vi "Event Camera.vi"() -> ()   [LabVIEW 2025]
panel:
  in  "Stop Preview":bool
  out "Image":T1(plugin-control)
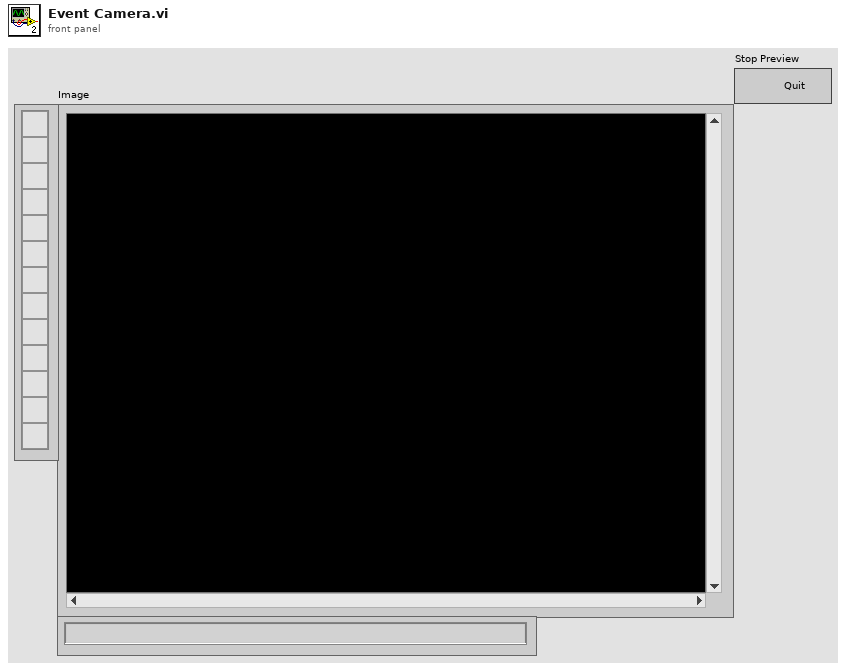
[diagram p1: front panel]
types:
  T1 = typedef "IMAQ Image.ctl" = refnum<image>
  T2 = typedef "Image Type" = u32
  T3 = enum16{"open", "replace", "create", "open or create", "replace or create", "replace or create with confirmation"}
  T4 = enum16{"big-endian, network order", "native, host order", "little-endian"}
  T5 = enum16{"Standard", "Buffered", "CRLF", "Immediate"}
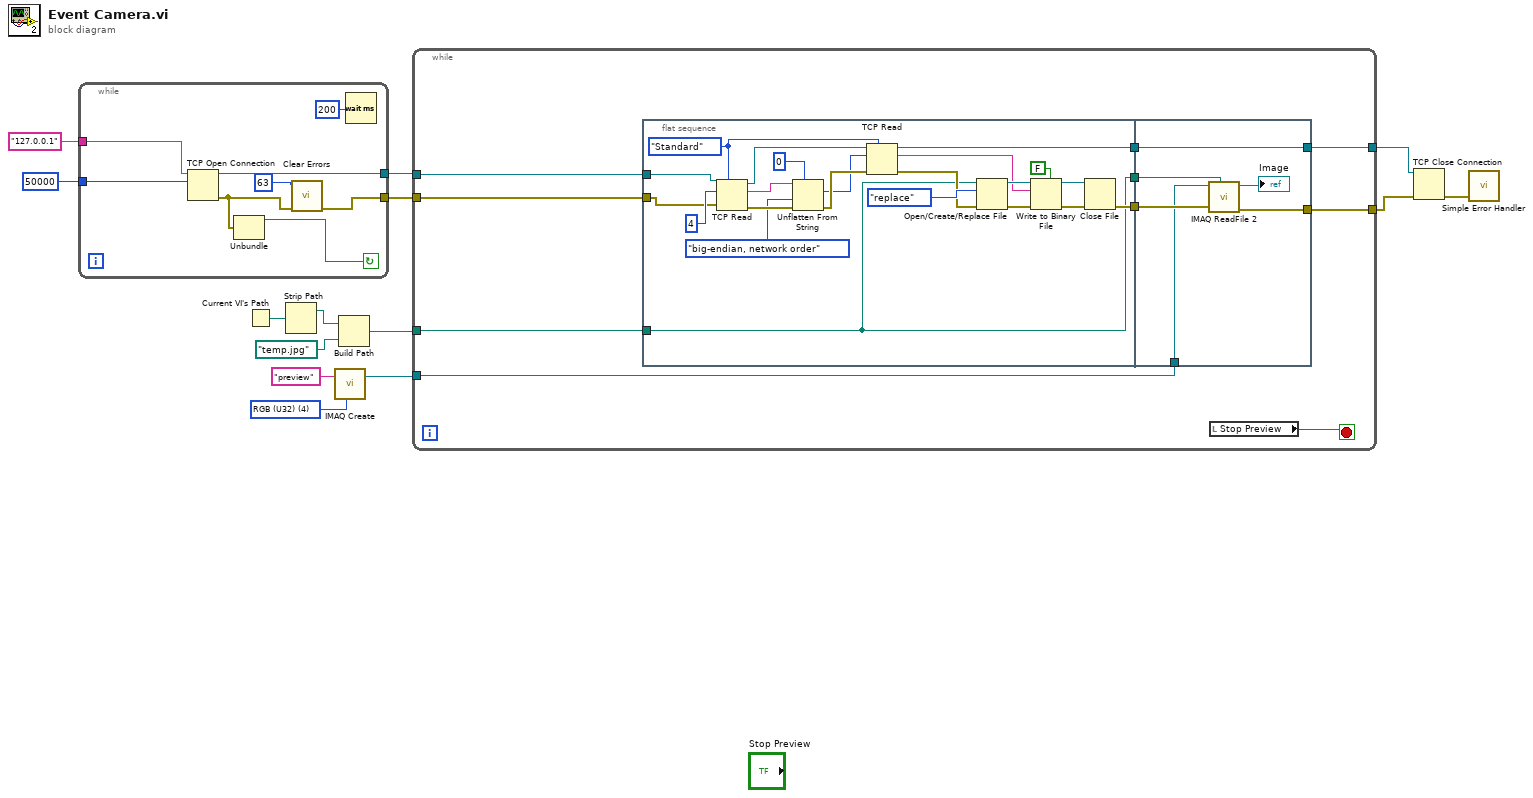
[diagram p0: block diagram]
diagram:
  w10 = T2 4 items=["Grayscale (U8)", "Grayscale (I16)", "Grayscale (SGL)", "Complex (CSG)", "RGB (U32)", "HSL (U32)", "RGB (U64)", "Grayscale (U16)"] ("Image Type")
  n1 = while {
    tunnel: [w19] -> w11
    tunnel: [w22] -> w12
    tunnel: u16 50000 ("remote port or service name") -> [w21]
    tunnel: "127.0.0.1" ("address") -> [w15]
    stop <- w16 continue-if-true
    n2 = TCP Open Connection(address=w15, remote port or service name=w21) -> (connection ID=w22:refnum<k5>, error out=w20:errorcluster)  [unwired: 3 in]
    n3 = Unbundle(w20) -> ("status"=w16:bool)  [unwired: 2 out]
    n4 = call <vilib>:"Clear Errors.vi"("error in (no error)"=w20, "specific error code to clear (0: all)"=63) -> ("error out"=w19:errorcluster)  [unwired: 4 in, 1 out]
    n5 = Wait (ms)(milliseconds to wait=u32 200) -> ()  [unwired: 1 out]
  }
  n6 = Current VI's Path() -> (path=w2:path)
  n7 = Strip Path(path=w2) -> (stripped path=w1:path)  [unwired: 1 out]
  n8 = call "IMAQ Create"("Image Name"="preview", "Image Type"=w10) -> ("New Image"=w6:T1)  [unwired: 3 in, 1 out]
  n9 = Build Path(base path=w1, name or relative path=path "temp.jpg") -> (appended path=w3:path)
  n10 = while {
    tunnel: w6 -> [w27]
    tunnel: [w28] -> w5
    tunnel: [w32] -> w4
    tunnel: w3 -> [w30]
    tunnel: w11 -> [w25]
    tunnel: w12 -> [w24]
    stop <- w23 stop-if-true
    n11 = flat-sequence {
      tunnel: w30 -> [w36]
      tunnel: [w38] -> w31
      tunnel: [w37] -> w29
      tunnel: [w36] -> w26
      tunnel: w25 -> [w34]
      tunnel: w24 -> [w33]
      tunnel: [w60] -> w32
      tunnel: w31 -> [w60]
      tunnel: w29 -> [w59]
      tunnel: [w58] -> w28
      tunnel: w27 -> [w57]
      tunnel: w26 -> [w56]
      frame #0 {
        w47 = T5."Standard" ("mode (standard)")
        n12 = TCP Read(connection ID=w33, bytes to read=4, error in (no error)=w34, 7:w47) -> (connection ID out=w50:refnum<k5>, data out=w35:string, error out=w53:errorcluster)  [unwired: 1 in]
        n13 = Unflatten From String(type=0, binary string=w35, byte order (0:big-endian, network order)=T4."big-endian, network order", error in (no error)=w53) -> (value=w48:i32, error out=w49:errorcluster)  [unwired: 1 in, 1 out]
        n14 = TCP Read(connection ID=w50, bytes to read=w48, error in (no error)=w49, 7:w47) -> (connection ID out=w38:refnum<k5>, data out=w43:string, error out=w45:errorcluster)  [unwired: 1 in]
        n15 = Open/Create/Replace File(file path (use dialog)=w36, error in=w45, operation (0:open)=T3."replace") -> (refnum out=w44:refnum<file>, error out=w41:errorcluster)  [unwired: 3 in, 1 out]
        n16 = Write to Binary File(file (use dialog)=w44, data=w43, error in=w41, 5:FALSE ("prepend array or string size? (T)")) -> (refnum out=w39:refnum<file>, error out=w40:errorcluster)  [unwired: 2 in, 1 out]
        n17 = Close File(refnum=w39, error in=w40) -> (error out=w37:errorcluster)  [unwired: 1 out]
      }
      frame #1 {
        n18 = call "IMAQ ReadFile 2"("File Path"=w56, "error in (no error)"=w59, "Image"=w57) -> ("error out"=w58:errorcluster, "Image Out"=→"Image":T1)  [unwired: 4 in, 3 out]
      }
    }
    n19 = local read "Stop Preview"() -> (w23:bool)
  }
  n20 = TCP Close Connection(connection ID=w4, error in (no error)=w5) -> (error out=w7:errorcluster)  [unwired: 1 in, 1 out]
  n21 = call <vilib>:"Simple Error Handler.vi"("error in (no error)"=w7) -> ()  [unwired: 4 in, 5 out]
